vi "accelerometer_transform.vi"() -> (2 "ASAP to Surface rotation":T1)   [LabVIEW 2013]
uses:
  <vilib>/Analysis/NI_AALBase.lvlib
  <vilib>/Analysis/baseanly.llb/Real A x B.vi
  <vilib>/Analysis/Matrix/NI_Matrix.lvlib
  <vilib>/Analysis/Matrix/Numeric/Conversions/Matrix To Array - RM.vi
  <vilib>/Analysis/NI_AALPro.lvlib
  <vilib>/Analysis/_algsub.llb/Real Vector Norm.vi
  <vilib>/Analysis/Matrix/Numeric/Subtract/Subtract - RM,RM.vi
  <vilib>/Analysis/Matrix/Numeric/Conversions/Array To Matrix - RA2.vi
  <vilib>/Analysis/3filter.llb/Butterworth Filter (DBL).vi
  <vilib>/Analysis/baseanly.llb/Mean (DBL).vi
  <vilib>/Analysis/Matrix/Datatypes/RealMatrix.ctl
panel:
  in  "Numeric 2":dbl=-0.77
  out "Raw Accelerometer Data":dbl[][](array[numeric])=[[-0.000224892, -0.000831316, -0.000165054]]
  in  "Filter Data":bool=TRUE
  out "Filtered Accelerometer Data":dbl[][](array[numeric])=[[-0.000224892, -0.000831316, -0.000165054]]
  in  "World z axis":dbl[](array[numeric])=[0.0, 0.0, 1.0]
  in  "Accelerometer Zero":T1=[[2.573711535990242, 2.526860047906293, 2.532033022687197]]
  in  "Accelerometer Mag":dbl=0.974868615762967
  in  "Surface Normal":dbl[][](array[numeric])=[[0.0, 0.0, 1.0]]
  # "Currently  configured for accepting input from the CXL02LF3 accelerometer.\nThe current calculation  assumes the surface normal to be defined by the\ngravity vector from the accelerometer\n\nData is filtered with a 2nd order lowpass butterworth with fl: 5 and fh: 30"
  # "Parameters:"
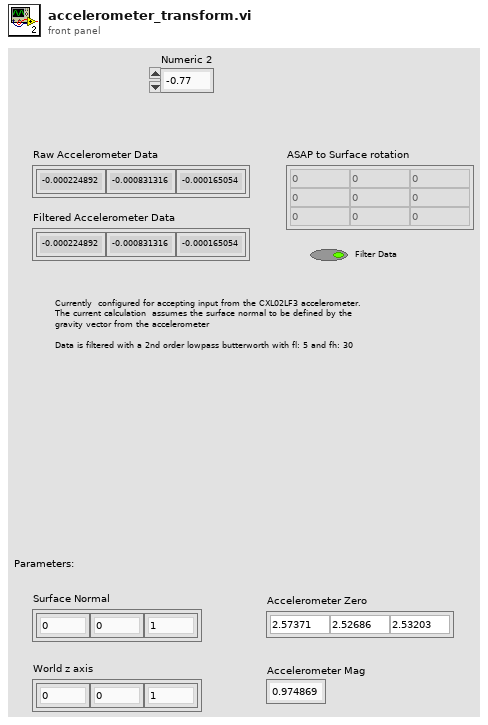
[diagram p1: front panel]
types:
  T1 = typedef "NI_Matrix.lvlib/RealMatrix.ctl" = dbl[][]
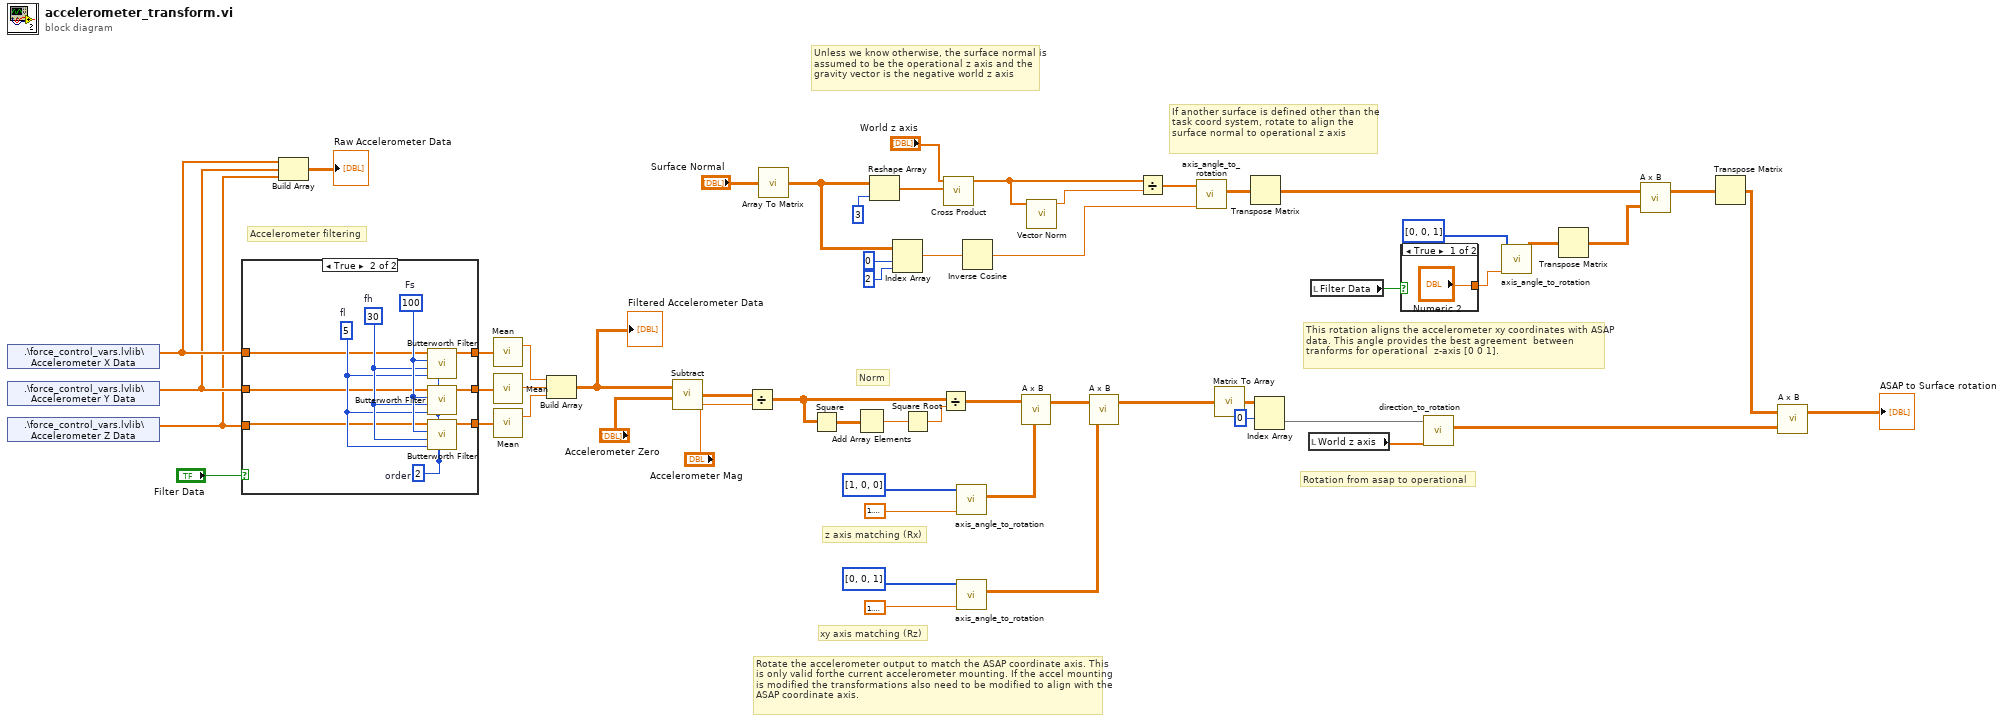
[diagram p0: block diagram]
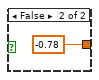
[diagram p2: hidden frame]
diagram:
  # "Norm"
  # "Accelerometer filtering"
  # "This rotation aligns the accelerometer xy coordinates with ASAP data. This angle provides the best agreement  between tranforms for operational  z-axis [0 0 1]."
  # "Unless we know otherwise, the surface normal is assumed to be the operational z axis and the gravity vector is the negative world z axis"
  # "xy axis matching (Rz)"
  # "z axis matching (Rx)"
  # "Rotate the accelerometer output to match the ASAP coordinate axis. This is only valid forthe current accelerometer mounting. If the accel mounting is modified the transformations also need to be modified to align with the ASAP coordinate axis."
  # "Rotation from asap to operational"
  # "If another surface is defined other than the task coord system, rotate to align the surface normal to operational z axis"
  n1 = shared-variable ".\\force_control_vars.lvlib\\Accelerometer X Data"() -> (w15:dbl[])  [unwired: 1 in, 1 out]
  n2 = shared-variable ".\\force_control_vars.lvlib\\Accelerometer Y Data"() -> (w14:dbl[])  [unwired: 1 in, 1 out]
  n3 = shared-variable ".\\force_control_vars.lvlib\\Accelerometer Z Data"() -> (w13:dbl[])  [unwired: 1 in, 1 out]
  n4 = case shown="True" "Filter Data" {
    tunnel: [w57 w64] -> w24
    tunnel: [w58 w63] -> w23
    tunnel: [w56 w62] -> w22
    tunnel: w15 -> [w57 w61]
    tunnel: w14 -> [w58 w60]
    tunnel: w13 -> [w56 w59]
    frame False {
    }
    frame True {
      w65 = 5  # fl
      w66 = 30  # fh
      w67 = 100  # Fs
      w68 = 2  # order
      n5 = call-poly <vilib>:"Butterworth Filter.vi"("order"=w68, "low cutoff freq: fl"=w65, "high cutoff freq: fh"=w66, "sampling freq: fs"=w67, "X"=w61) -> ("Filtered X"=w64:dbl[])  [unwired: 3 in, 1 out]
      n6 = call-poly <vilib>:"Butterworth Filter.vi"("order"=w68, "low cutoff freq: fl"=w65, "high cutoff freq: fh"=w66, "sampling freq: fs"=w67, "X"=w60) -> ("Filtered X"=w63:dbl[])  [unwired: 3 in, 1 out]
      n7 = call-poly <vilib>:"Butterworth Filter.vi"("order"=w68, "low cutoff freq: fl"=w65, "high cutoff freq: fh"=w66, "sampling freq: fs"=w67, "X"=w59) -> ("Filtered X"=w62:dbl[])  [unwired: 3 in, 1 out]
    }
  }
  n8 = Build Array(w15, w14, w13) -> (→"Raw Accelerometer Data":T1)
  n9 = call-poly <vilib>:"Mean.vi"("X"=w24) -> ("mean"=w21:dbl)  [unwired: 1 out]
  n10 = call-poly <vilib>:"Mean.vi"("X"=w23) -> ("mean"=w20:dbl)  [unwired: 1 out]
  n11 = call-poly <vilib>:"Mean.vi"("X"=w22) -> ("mean"=w19:dbl)  [unwired: 1 out]
  n12 = Build Array(w21, w20, w19) -> (w17:T1)
  "Filtered Accelerometer Data" <- w17
  n13 = call-poly <vilib>:"Subtract.vi"("Real Matrix B"="Accelerometer Zero", "Real Matrix A"=w17) -> ("A - B"=w40:T1)
  n14 = Divide(x=w40, y="Accelerometer Mag") -> (x/y=w28:T1)
  n15 = call-poly <vilib>:"Array To Matrix.vi"("Real 2D Array"="Surface Normal") -> ("Real Matrix"=w25:T1)
  n16 = Square(x=w28) -> (x^2=w30:T1)
  n17 = Add Array Elements(numeric array=w30) -> (sum=w29:dbl)
  n18 = Reshape Array(w25, 3) -> (w53:dbl[])
  n19 = Index Array(array=w25, index (row)=0, index (col)=2) -> (element=w48:dbl)
  n20 = Square Root ("Square Root.vi")(x=w29) -> (sqrt(x)=w27:dbl)
  n21 = Divide(x=w28, y=w27) -> (x/y=w10:T1)
  n22 = call <vilib>:"Cross Product.vi"("B Vector"=w53, "A Vector"="World z axis") -> ("Cross Product"=w47:dbl[])  [unwired: 8 in, 1 out]
  n23 = call "axis_angle_to_rotation.vi"("Angle"=1.5707963267948966, "Axis"=i32[] [1, 0, 0]) -> ("Rotation"=w37:T1)  [unwired: 9 in]
  n24 = call "axis_angle_to_rotation.vi"("Angle"=1.5707963267948966, "Axis"=i32[] [0, 0, 1]) -> ("Rotation"=w35:T1)  [unwired: 9 in]
  n25 = Inverse Cosine(1:w48) -> (0:w45:dbl)
  n26 = call-poly <vilib>:"A x B.vi"("B"=w37, "A"=w10) -> ("A x B"=w36:T1)  [unwired: 1 out]
  n27 = call-poly <vilib>:"Vector Norm.vi"("Input Vector"=w47) -> ("norm"=w52:dbl)  [unwired: 9 in, 1 out]
  n28 = call-poly <vilib>:"A x B.vi"("B"=w35, "A"=w36) -> ("A x B"=w6:T1)  [unwired: 1 out]
  n29 = Divide(x=w47, y=w52) -> (x/y=w46:dbl[])
  n30 = call "axis_angle_to_rotation.vi"("Angle"=w45, "Axis"=w46) -> ("Rotation"=w44:T1)  [unwired: 9 in]
  n31 = call-poly <vilib>:"Matrix To Array.vi"("Real Matrix"=w6) -> ("Real 2D Array"=w9:dbl[][])
  n32 = Transpose Matrix(1:w44) -> (0:w41:T1)
  n33 = Index Array(array=w9, index (row)=0) -> (element=w4:dbl[])  [unwired: 1 in]
  n34 = local read "World z axis"() -> (w5:dbl[])
  n35 = local read "Filter Data"() -> (w11:bool)
  n36 = case shown="True" w11 {
    tunnel: ["Numeric 2" -0.78 ("Numeric")] -> w12
    frame True {
    }
    frame False {
    }
  }
  n37 = call "direction_to_rotation.vi"("To"=w5, "From"=w4) -> ("Rotation"=w1:T1)  [unwired: 9 in]
  n38 = call "axis_angle_to_rotation.vi"("Angle"=w12, "Axis"=i32[] [0, 0, 1]) -> ("Rotation"=w54:T1)  [unwired: 9 in]
  n39 = Transpose Matrix(1:w54) -> (0:w43:T1)
  n40 = call-poly <vilib>:"A x B.vi"("B"=w43, "A"=w41) -> ("A x B"=w3:T1)  [unwired: 1 out]
  n41 = Transpose Matrix(1:w3) -> (0:w42:T1)
  n42 = call-poly <vilib>:"A x B.vi"("B"=w1, "A"=w42) -> ("A x B"=→"ASAP to Surface rotation":T1)  [unwired: 1 out]
